vi "mat_display_grayscale.vi"() -> ()   [LabVIEW 2015]
uses:
  <vilib>/imath/engines/lvmath2/RunTimeEngine/BuiltInFunctions/view_image/NIMS_view_image.vi
  <vilib>/imathl/engines/lvmath/Functions/Error Handling/Create Error.vi
  <vilib>/imath/engines/lvmath2/RunTimeEngine/ErrorHandling/NIMS_Finalize Error.vi
  <vilib>/picture/picture.llb/Draw 4-Bit Pixmap.vi
panel:
  out "new picture":picture
  out "Array":i32[][](array[numeric])
  out "output 2":i32
  out "output 1":i32
  in  "Path 7":path
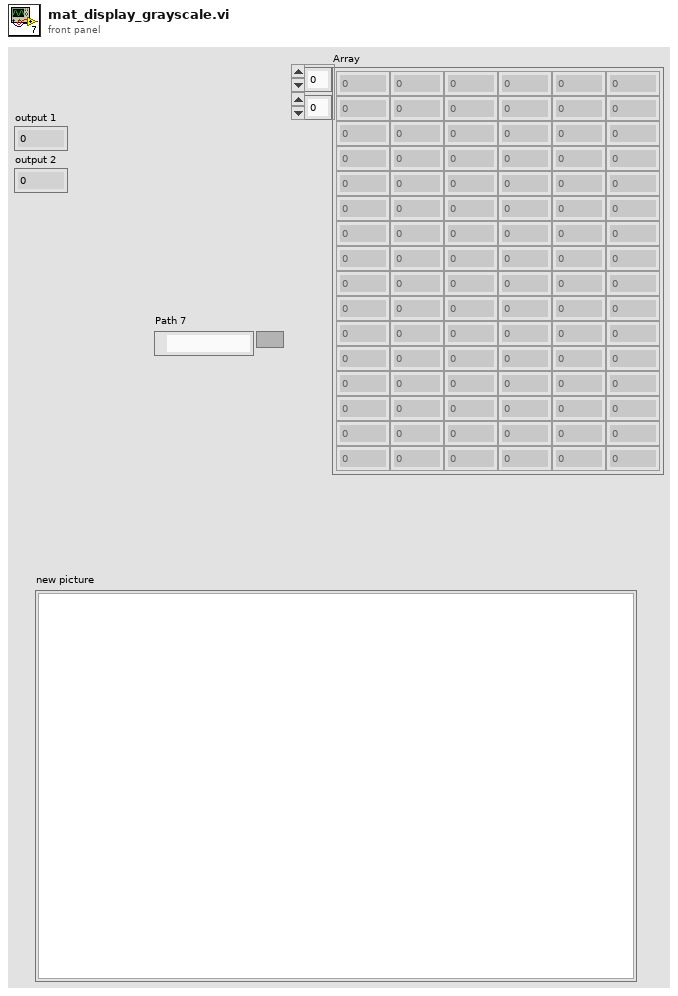
[diagram p1: front panel]
types:
  T1 = enum16{"open", "replace", "create", "open or create", "replace or create", "replace or create with confirmation"}
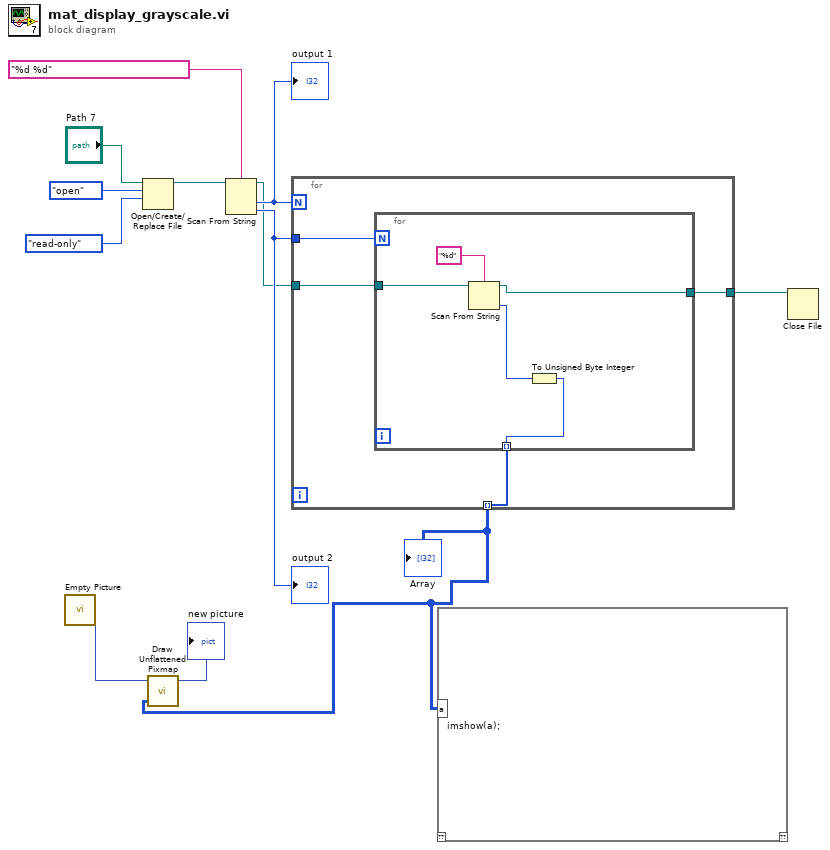
[diagram p0: block diagram]
diagram:
  n1 = call "Empty Picture"() -> ("empty picture"=w3:picture)
  n2 = Open/Create/Replace File(file path (use dialog)="Path 7", operation (0:open)=T1."open", access (0:read/write)=enum16{"read/write", "read-only", "write-only"}."read-only") -> (refnum out=w9:refnum<file>)  [unwired: 3 in, 2 out]
  n3 = Scan From String("%d %d" ("format string"), w9) -> (w5:refnum<file>, output 1=w7:i32, output 2=w6:i32)  [unwired: 3 in, 1 out]
  "output 1" <- w7
  "output 2" <- w6
  n4 = for {
    N: w7 -> [_]
    tunnel: w6 -> [w16]
    tunnel: w5 -> [w15]
    tunnel: [w14] -> w2 mode=indexing
    tunnel: [w13] -> w4
    n5 = for {
      N: w16 -> [_]
      tunnel: w15 -> [w21]
      tunnel: [w17] -> w14 mode=indexing
      tunnel: [w19] -> w13
      n6 = Scan From String("%d" ("format string"), w21) -> (w19:refnum<file>, output 1=w18:i32)  [unwired: 2 in, 1 out]
      n7 = To Unsigned Byte Integer(number=w18) -> (unsigned 8bit integer=w17:u8)
    }
  }
  "Array" <- w2
  n8 = call-poly <vilib>:"Draw Unflattened Pixmap.vi"("picture"=w3, "data"=w2) -> ("new picture"=→"new picture":picture)  [unwired: 7 in]
  n9 = mathscript code="imshow(a);"("a"=w2) -> ()  [unwired: 1 in, 1 out]
  n10 = Close File(refnum=w4) -> ()  [unwired: 1 in, 2 out]
